vi "Get Server Command Specifier.vi"(8 "error in":errorcluster, 11 "CANopen Response in":refnum<class "CANopen Response Message.lvclass">) -> (0 "error out":errorcluster, 2 "Server Command Specifier":T1, 3 "CANopen Response out":refnum<class "CANopen Response Message.lvclass">)   [LabVIEW 2024, in "CANopen Master.lvlib" / "CANopen Response Message.lvclass"]
uses:
  CANopen Response Message.lvclass
  CANopen 2/Server Command Specifier.ctl
  CANopen Message/CANopen Message.lvclass/CANopen Message.ctl
  CANopen Message/CANopen Message.lvclass
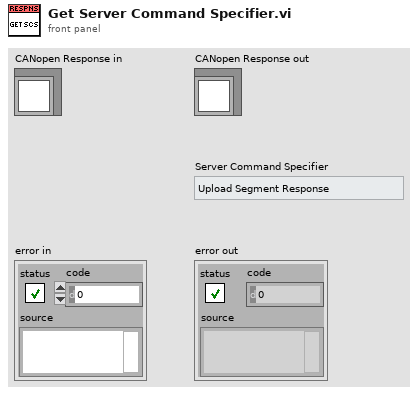
[diagram p1: front panel]
types:
  T1 = typedef "CANopen Master.lvlib/CANopen Response Message.lvclass/Server Command Specifier.ctl" = enum8{"Upload Segment Response", "Download Segment Response", "Initiate Upload Response", "Initiate Download Response", "Heartbeat", "Block Download"}
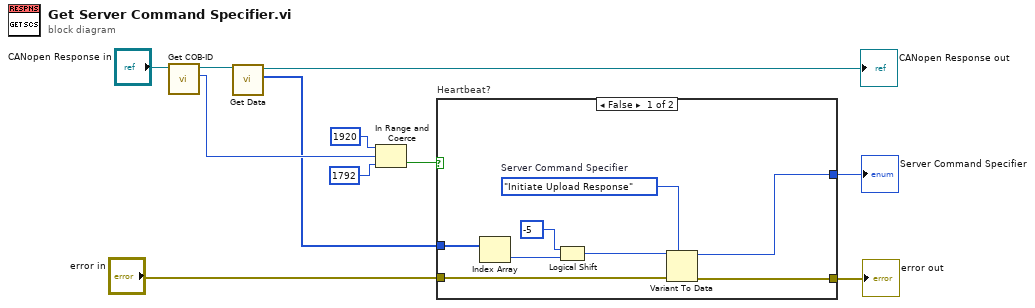
[diagram p0: block diagram]
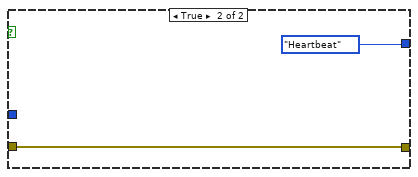
[diagram p2: hidden frame]
diagram:
  n1 = call "Get COB-ID.vi"("CANopen Message in"="CANopen Response in") -> ("COB-ID"=w2:u32, "CANopen Message out"=w7:refnum<class "CANopen Response Message.lvclass">)  [unwired: 9 in]
  n2 = call "Get Data.vi"("CANopen Message in"=w7) -> ("Data"=w1:u8[], "CANopen Message out"=→"CANopen Response out":refnum<class "CANopen Response Message.lvclass">)  [unwired: 9 in]
  n3 = In Range and Coerce(upper limit=u32 1920 ("x"), x=w2, lower limit=u32 1792 ("x")) -> (In Range?=w9:bool)  [unwired: 1 out]
  n4 = case "Heartbeat?" shown="False" w9 {
    tunnel: w1 -> [w19 _]
    tunnel: "error in" -> [w14 w21]
    tunnel: [w13 w21] -> w4
    tunnel: [w12 Server_Command_Specifier."Heartbeat" ("Msg-Type")] -> w3
    frame False {
      w16 = Server_Command_Specifier."Initiate Upload Response"  # Server Command Specifier
      n5 = Index Array(array=w19) -> (element=w17:u8)  [unwired: 1 in]
      n6 = Logical Shift(y=-5 ("x"), x=w17) -> (x << y=w15:u8)
      n7 = Variant To Data(error in=w14, type=w16, Variant=w15) -> (data=w12:T1, error out=w13:errorcluster)
    }
    frame True {
    }
  }
  "error out" <- w4
  "Server Command Specifier" <- w3
